vi "RenderRobotPose.vi"(4 "Reset":bool, 5 "Buffer Time (min)":dbl=5.0 format="%#_13g", 6 "Robot Enabled":bool, 7 "Robot Size (in)":dbl=30.0 format="%#_13g", 8 "Turret Heading (deg)":dbl, 9 "Robot Heading (deg)":dbl, 10 "Robot Y (in)":dbl, 11 "Robot X (in)":dbl) -> (2 "Robot Pose":cluster{dbl[], dbl[]}[](array[cluster]))   [LabVIEW 2019]
doc: "This VI takes the robot pose information as input and renders a plot to display it. At this time, only square robot dimensions are supported."
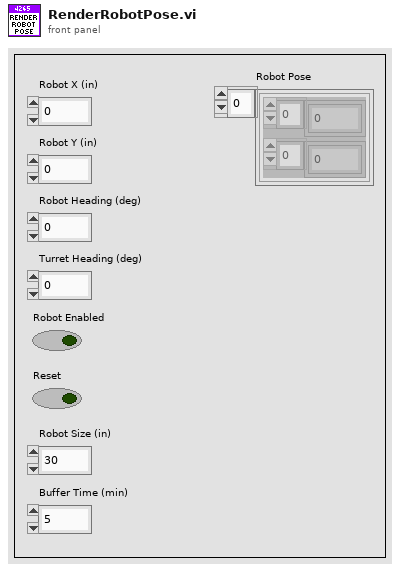
[diagram p1: front panel]
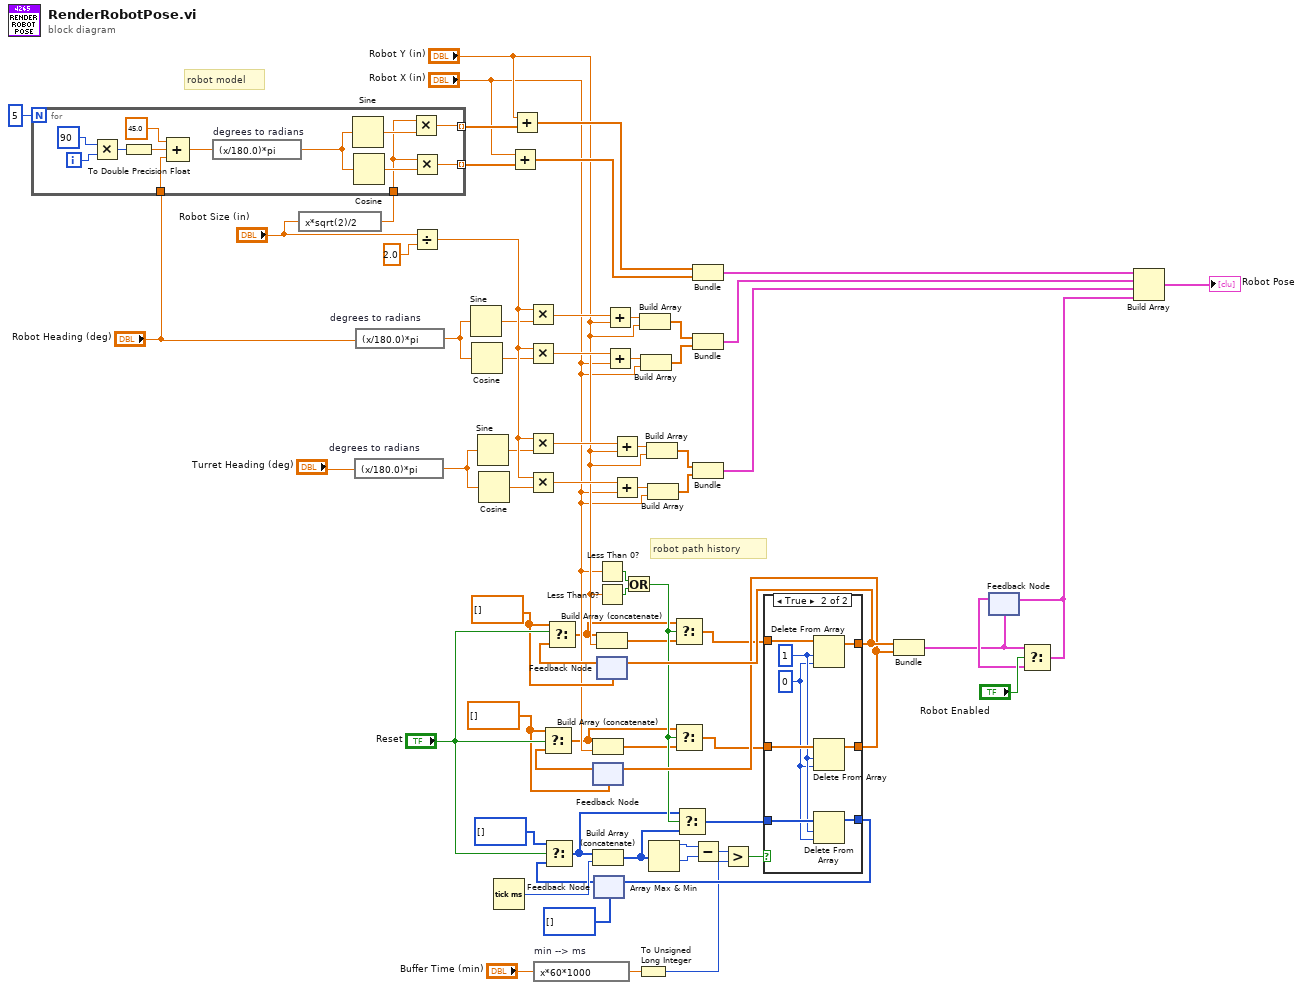
[diagram p0: block diagram]
diagram:
  w13 = dbl[] [] ("t")
  w12 = dbl[] [] ("t")
  # "robot model"
  # "robot path history"
  n1 = expression code="x*sqrt(2)/2"("Robot Size (in)") -> (w69:dbl)
  n2 = for {
    N: 5 -> [_]
    tunnel: [w80] -> w65 mode=indexing
    tunnel: [w79] -> w64 mode=indexing
    tunnel: "Robot Heading (deg)" -> [w73]
    tunnel: w69 -> [w71]
    i -> [w78]
    n3 = Multiply(x=90, y=w78) -> (x*y=w76:i32)
    n4 = To Double Precision Float(number=w76) -> (double precision float=w75:dbl)
    n5 = Compound Arithmetic op=ADD(45.0 ("value"), w75, w73) -> (w74:dbl)
    n6 = expression code="(x/180.0)*pi" "degrees to radians"(w74) -> (w82:dbl)
    n7 = Sine(x=w82) -> (sin(x)=w81:dbl)
    n8 = Cosine(x=w82) -> (cos(x)=w83:dbl)
    n9 = Multiply(x=w71, y=w81) -> (x*y=w79:dbl)
    n10 = Multiply(x=w71, y=w83) -> (x*y=w80:dbl)
  }
  n11 = expression code="(x/180.0)*pi" "degrees to radians"("Turret Heading (deg)") -> (w39:dbl)
  n12 = expression code="(x/180.0)*pi" "degrees to radians"("Robot Heading (deg)") -> (w28:dbl)
  n13 = Divide(x="Robot Size (in)", y=2.0) -> (x/y=w67:dbl)
  n14 = Sine(x=w28) -> (sin(x)=w27:dbl)
  n15 = Cosine(x=w28) -> (cos(x)=w26:dbl)
  n16 = Sine(x=w39) -> (sin(x)=w38:dbl)
  n17 = Cosine(x=w39) -> (cos(x)=w37:dbl)
  n18 = Tick Count (ms)() -> (millisecond timer value=w46:u32)
  n19 = Add(x="Robot X (in)", y=w65) -> (x+y=w62:dbl[])
  n20 = Add(x="Robot Y (in)", y=w64) -> (x+y=w61:dbl[])
  n21 = Multiply(x=w67, y=w27) -> (x*y=w25:dbl)
  n22 = Multiply(x=w67, y=w26) -> (x*y=w24:dbl)
  n23 = Multiply(x=w67, y=w38) -> (x*y=w36:dbl)
  n24 = Multiply(x=w67, y=w37) -> (x*y=w35:dbl)
  n25 = expression code="x*60*1000" "min --> ms"("Buffer Time (min)") -> (w52:dbl)
  n26 = feedback #1(w12) -> (w42:dbl[])
  n27 = Select(t=w12, s="Reset", f=w42) -> (s? t:f=w1:dbl[])
  n28 = Build Array (concatenate)(w1, "Robot X (in)") -> (w2:dbl[])
  n29 = feedback #2(u32[] []) -> (w44:u32[])
  n30 = Select(t=u32[] [], s="Reset", f=w44) -> (s? t:f=w6:u32[])
  n31 = Build Array (concatenate)(w6, w46) -> (w5:u32[])
  n32 = Less Than 0?(x="Robot X (in)") -> (x < 0?=w9:bool)
  n33 = Less Than 0?(x="Robot Y (in)") -> (x < 0?=w10:bool)
  n34 = feedback #3(w13) -> (w45:dbl[])
  n35 = Select(t=w13, s="Reset", f=w45) -> (s? t:f=w3:dbl[])
  n36 = Build Array (concatenate)(w3, "Robot Y (in)") -> (w4:dbl[])
  n37 = Add(x=w25, y="Robot Y (in)") -> (x+y=w23:dbl)
  n38 = Add(x=w24, y="Robot X (in)") -> (x+y=w22:dbl)
  n39 = Add(x=w36, y="Robot Y (in)") -> (x+y=w34:dbl)
  n40 = Add(x=w35, y="Robot X (in)") -> (x+y=w33:dbl)
  n41 = Or(x=w9, y=w10) -> (x .or. y?=w8:bool)
  n42 = To Unsigned Long Integer(number=w52) -> (unsigned 32bit integer=w53:u32)
  n43 = Build Array(w23, "Robot Y (in)") -> (w21:dbl[])
  n44 = Build Array(w22, "Robot X (in)") -> (w20:dbl[])
  n45 = Build Array(w34, "Robot Y (in)") -> (w32:dbl[])
  n46 = Build Array(w33, "Robot X (in)") -> (w31:dbl[])
  n47 = Array Max & Min(array=w5) -> (max value=w49:u32, min value=w50:u32)  [unwired: 2 out]
  n48 = Select(t=w3, s=w8, f=w4) -> (s? t:f=w15:dbl[])
  n49 = Select(t=w1, s=w8, f=w2) -> (s? t:f=w14:dbl[])
  n50 = Select(t=w6, s=w8, f=w5) -> (s? t:f=w7:u32[])
  n51 = Bundle(w61, w62) -> (w30:cluster{dbl[], dbl[]})  [unwired: 1 in]
  n52 = Bundle(w21, w20) -> (w29:cluster{dbl[], dbl[]})  [unwired: 1 in]
  n53 = Bundle(w32, w31) -> (w40:cluster{dbl[], dbl[]})  [unwired: 1 in]
  n54 = Subtract(x=w49, y=w50) -> (x-y=w51:u32)
  n55 = Greater?(x=w51, y=w53) -> (0:w55:bool)
  n56 = case shown="True" w55 {
    tunnel: w7 -> [w84 w92]
    tunnel: w14 -> [w85 w93]
    tunnel: w15 -> [w86 w94]
    tunnel: [w86 w89] -> w58
    tunnel: [w85 w88] -> w57
    tunnel: [w84 w87] -> w56
    frame False {
    }
    frame True {
      w90 = 0 ("index")
      w91 = 1 ("length")
      n57 = Delete From Array(array=w94, length=w91, index=w90) -> (array with subset deleted=w89:dbl[])  [unwired: 1 out]
      n58 = Delete From Array(array=w93, length=w91, index=w90) -> (array with subset deleted=w88:dbl[])  [unwired: 1 out]
      n59 = Delete From Array(array=w92, length=w91, index=w90) -> (array with subset deleted=w87:u32[])  [unwired: 1 out]
    }
  }
  n60 = feedback-in #1(w57) -> ()
  n61 = feedback-in #2(w56) -> ()
  n62 = feedback-in #3(w58) -> ()
  n63 = Bundle("t"=w58, "t"=w57) -> (w18:cluster{"t":dbl[], "t":dbl[]})  [unwired: 1 in]
  n64 = feedback #4(w18) -> (w59:cluster{"t":dbl[], "t":dbl[]})
  n65 = Select(t=w18, s="Robot Enabled", f=w59) -> (s? t:f=w17:cluster{"t":dbl[], "t":dbl[]})
  n66 = feedback-in #4(w17) -> ()
  n67 = Build Array(w30, w29, w40, w17) -> (→"Robot Pose":cluster{"t":dbl[], "t":dbl[]}[])
